vi "Split to Multiline String.vi"(1 "Line Index":i32, 2 "Delimiter":string, 3 "Singleline String":string) -> (0 "Multiline String":string)   [LabVIEW 2019]
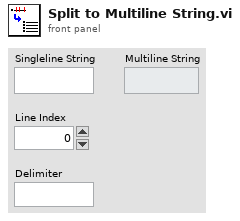
[diagram p1: front panel]
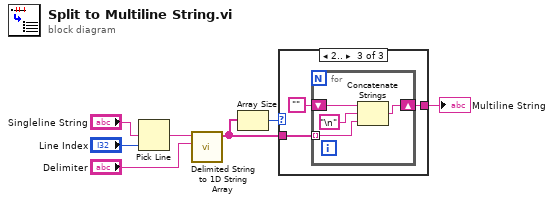
[diagram p0: block diagram]
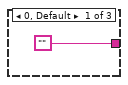
[diagram p2: hidden frame]
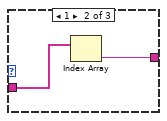
[diagram p3: hidden frame]
diagram:
  n1 = Pick Line(multi-line string="Singleline String", line index="Line Index") -> (output string=w3:string)  [unwired: 1 in]
  n2 = call <vilib>:"Delimited String to 1D String Array.vi"("delimiter"="Delimiter", "delimited string"=w3) -> ("string array"=w6:string[])  [unwired: 9 in]
  n3 = Array Size(array=w6) -> (size(s)=w5:i32)
  n4 = case shown="2.." w5 {
    tunnel: w6 -> [_ w10 w13]
    tunnel: ["" w9 w11] -> w7
    frame 0, Default {
    }
    frame 1 {
      n5 = Index Array(array=w10) -> (element=w9:string)  [unwired: 1 in]
    }
    frame 2.. {
      n6 = for {
        tunnel: w13 -> [w14] mode=indexing
        shift-right: [w17] -> w11
        shift-left: "" -> [w16]
        n7 = Concatenate Strings(w16, "\n", w14) -> (w17:string)
      }
    }
  }
  "Multiline String" <- w7
